vi "BT2_PluginConfig.vi"() -> (3 "Plugin list (output)":T1)   [LabVIEW 2011]
uses:
  BeadTracker2.llb/VisionExpressCamera.lvclass
  BeadTracker2.llb/CameraInterface.lvclass
  BeadTracker2.llb/MotorDriverInterface.lvclass
  BeadTracker2.llb/PluginConfig.ctl
panel:
  in  "Plugin List":T1
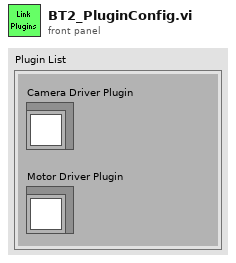
[diagram p1: front panel]
types:
  T1 = typedef "PluginConfig.ctl" = cluster{"Camera Driver Plugin":refnum<class "CameraInterface.lvclass">, "Motor Driver Plugin":refnum<class "MotorDriverInterface.lvclass">}
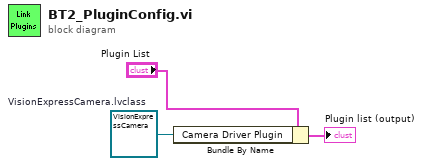
[diagram p0: block diagram]
diagram:
  w1 = refnum<class "VisionExpressCamera.lvclass"> refnum  # VisionExpressCamera.lvclass
  n1 = Bundle By Name(cluster="Plugin List", "Camera Driver Plugin"=w1) -> (→"Plugin list (output)":T1)
